vi "EOD Write Idea2.vi"(8 "EODDataInput":T1(array[cluster]), 11 "Number of Waveforms":i32) -> (0 "error out":errorcluster, 2 "Iteration Test":i32, 3 "refnum out":refnum<file>)   [LabVIEW 2014]
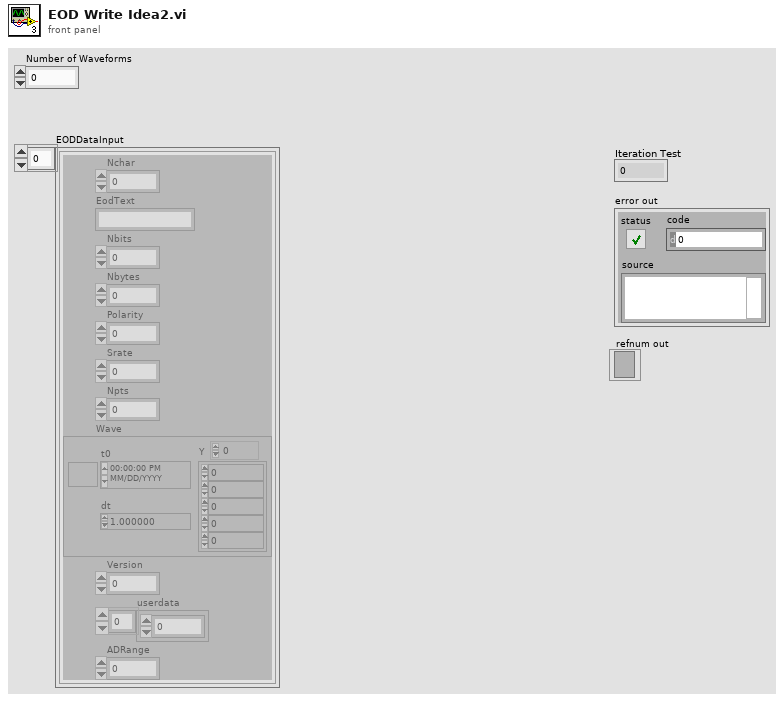
[diagram p1: front panel]
types:
  T1 = cluster{"Nchar":i32, "EodText":string, "Nbits":i32, "Nbytes":i32, "Polarity":i32, "Srate":i32, "Npts":i32, "Wave":waveform(dbl), "Version":i32, "userdata":dbl[], "ADRange":dbl}[]
  T2 = enum16{"open", "replace", "create", "open or create", "replace or create", "replace or create with confirmation"}
  T3 = enum16{"big-endian, network order", "native, host order", "little-endian"}
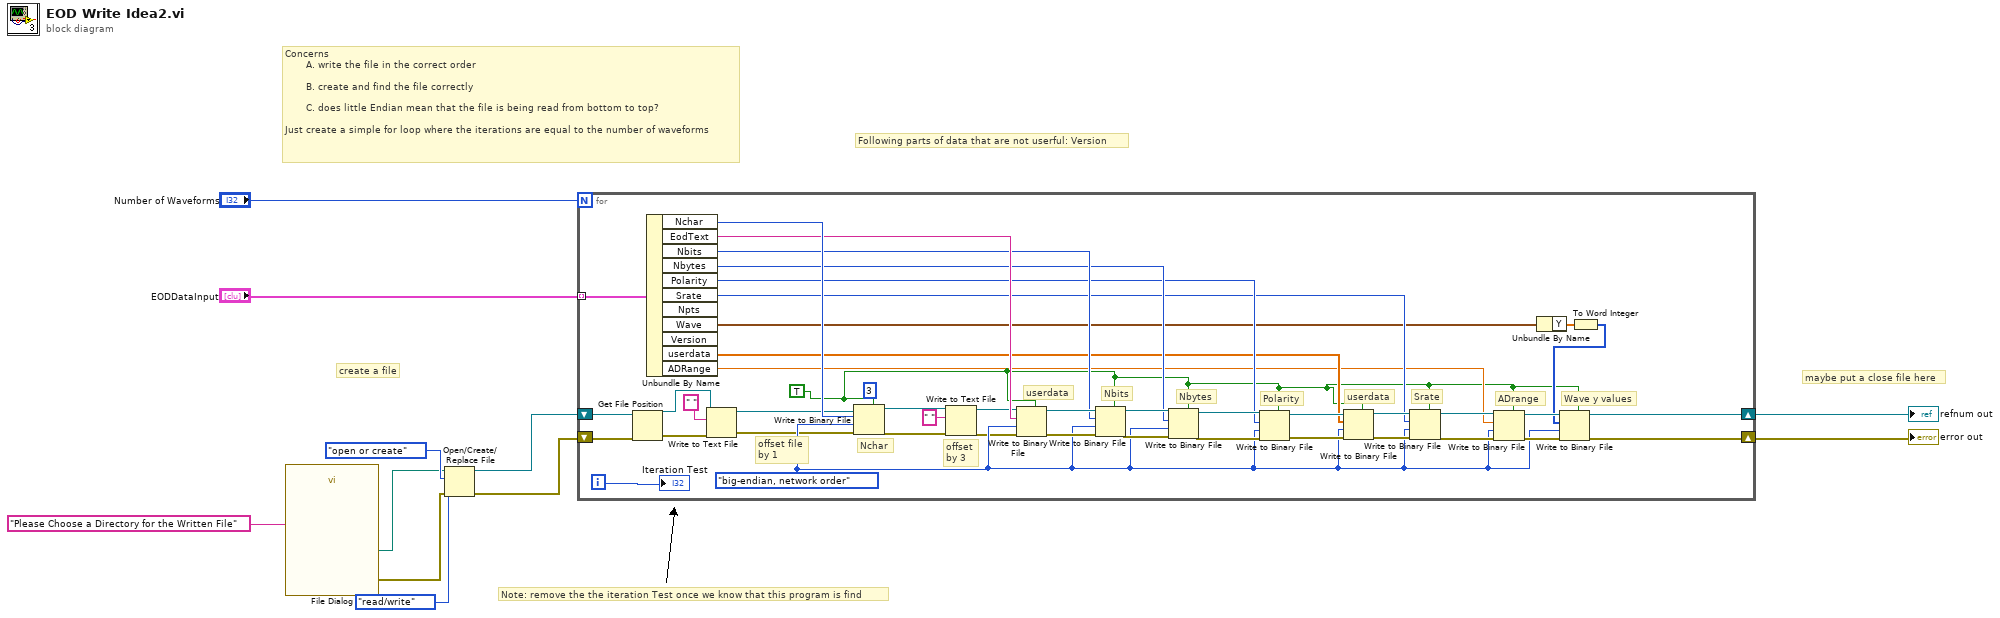
[diagram p0: block diagram]
diagram:
  # "maybe put a close file here"
  # "Note: remove the the iteration Test once we know that this program is find"
  # "Following parts of data that are not userful: Version"
  # "create a file"
  # "Concerns\n       A. write the file in the correct order\n\n       B. create and find the file correctly\n\n       C. does little Endian mean that the file is being read from bottom to top?\n\nJust create a simple for loop where the iterations are equal to the number of waveforms"
  n1 = call "File Dialog"("prompt"="Please Choose a Directory for the Written File") -> ("selected path"=w8:path, "error out"=w7:errorcluster)  [unwired: 11 in, 2 out]
  n2 = Open/Create/Replace File(file path (use dialog)=w8, error in=w7, operation (0:open)=T2."open or create", access (0:read/write)=enum16{"read/write", "read-only", "write-only"}."read/write") -> (refnum out=w5:refnum<file>, error out=w4:errorcluster)  [unwired: 2 in, 1 out]
  n3 = for {
    N: "Number of Waveforms" -> [_]
    tunnel: "EODDataInput" -> [w54] mode=indexing
    shift-right: [w28] -> w3
    shift-left: w5 -> [w27]
    shift-right: [w26] -> w2
    shift-left: w4 -> [w25]
    i -> [w23]
    w22 = TRUE
    (unwired) i64 3 ("y")
    w24 = T3."big-endian, network order" ("byte order (0:big-endian, network order)")
    # "Wave y values"
    # "ADrange"
    # "Srate"
    # "userdata"
    # "Polarity"
    # "Nbytes"
    # "offset\nby 3"
    # "offset file\nby 1"
    # "Nchar"
    # "Nbits"
    # "userdata"
    n4 = Get File Position(4:w25, 7:w27) -> (0:w20:errorcluster, 3:w17:refnum<file>)  [unwired: 1 out]
    n5 = Unbundle By Name(w54) -> ("Nchar"=w53:i32, "EodText"=w52:string, "Nbits"=w49:i32, "Nbytes"=w44:i32, "Polarity"=w43:i32, "Srate"=w37:i32, "Wave"=w33:waveform(dbl), "userdata"=w40:dbl[], "ADRange"=w34:dbl)  [unwired: 2 out]
    n6 = Write to Text File(file (use dialog)=w17, text=" ", error in=w20) -> (refnum out=w19:refnum<file>, error out=w18:errorcluster)  [unwired: 1 in, 1 out]
    n7 = Write to Binary File(file (use dialog)=w19, data=w53, error in=w18, 5:w22, 9:w24) -> (refnum out=w16:refnum<file>, error out=w13:errorcluster)  [unwired: 1 in, 1 out]
    n8 = Write to Text File(file (use dialog)=w16, text=" ", error in=w13) -> (refnum out=w15:refnum<file>, error out=w14:errorcluster)  [unwired: 1 in, 1 out]
    n9 = Write to Binary File(file (use dialog)=w15, data=w52, error in=w14, 5:w22, 9:w24) -> (refnum out=w51:refnum<file>, error out=w50:errorcluster)  [unwired: 1 in, 1 out]
    n10 = Write to Binary File(file (use dialog)=w51, data=w49, error in=w50, 5:w22, 9:w24) -> (refnum out=w48:refnum<file>, error out=w47:errorcluster)  [unwired: 1 in, 1 out]
    n11 = Write to Binary File(file (use dialog)=w48, data=w44, error in=w47, 5:w22, 9:w24) -> (refnum out=w46:refnum<file>, error out=w45:errorcluster)  [unwired: 1 in, 1 out]
    n12 = Write to Binary File(file (use dialog)=w46, data=w43, error in=w45, 5:w22, 9:w24) -> (refnum out=w42:refnum<file>, error out=w41:errorcluster)  [unwired: 1 in, 1 out]
    n13 = Write to Binary File(file (use dialog)=w42, data=w40, error in=w41, 5:w22, 9:w24) -> (refnum out=w39:refnum<file>, error out=w38:errorcluster)  [unwired: 1 in, 1 out]
    n14 = Write to Binary File(file (use dialog)=w39, data=w37, error in=w38, 5:w22, 9:w24) -> (refnum out=w36:refnum<file>, error out=w35:errorcluster)  [unwired: 1 in, 1 out]
    n15 = Write to Binary File(file (use dialog)=w36, data=w34, error in=w35, 5:w22, 9:w24) -> (refnum out=w31:refnum<file>, error out=w30:errorcluster)  [unwired: 1 in, 1 out]
    n16 = Unbundle By Name(w33) -> ("Y"=w32:dbl[])
    n17 = To Word Integer(number=w32) -> (16bit integer=w29:i16[])
    n18 = Write to Binary File(file (use dialog)=w31, data=w29, error in=w30, 5:w22, 9:w24) -> (refnum out=w28:refnum<file>, error out=w26:errorcluster)  [unwired: 1 in, 1 out]
    "Iteration Test" <- w23
  }
  "refnum out" <- w3
  "error out" <- w2
